vi "Move Motor.vi"(6 "Goal Speed (RPM)":dbl, 8 "error in (no error)":errorcluster, 9 "Goal Position (150 deg)":dbl=150.0 min=0.0 max=300.0, 10 "Motor ID (0)":u8, 11 "Dynamixel Motor Simulator in":refnum<class "Dynamixel Motor Simulator.lvclass">) -> (0 "error out":errorcluster, 3 "Dynamixel Motor Simulator out":refnum<class "Dynamixel Motor Simulator.lvclass">)   [LabVIEW 2016, in "Dynamixel Motor Simulator.lvclass"]
doc: "Sets the goal position for the motor."
uses:
  <instrlib>/Dynamixel Motor/HAIOL/Simulator/Dynamixel Motor Simulator.lvclass
  <instrlib>/Dynamixel Motor/HAIOL/Simulator/Dynamixel Motor Simulator.lvclass/Dynamixel Motor Simulator.ctl
  <vilib>/robotics/Simulator/Robot Factory/Motor/ODESimulator_Motor.lvclass
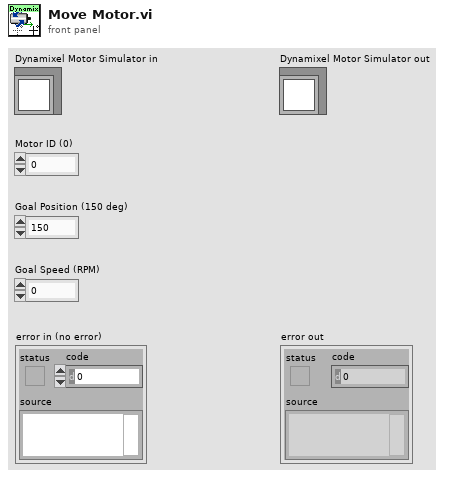
[diagram p1: front panel]
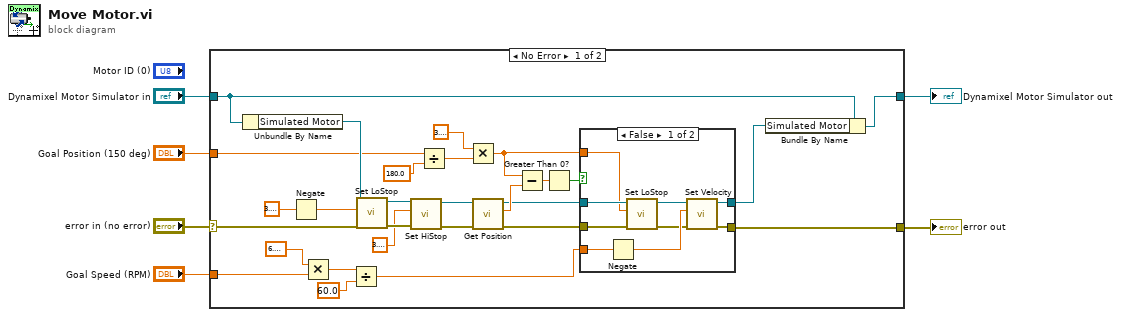
[diagram p0: block diagram]
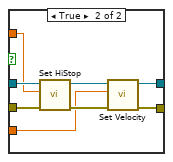
[diagram p2: hidden frame]
diagram:
  n1 = case shown="No Error" "error in (no error)" {
    selector: "error in (no error)" -> [w28 w52]
    tunnel: "Dynamixel Motor Simulator in" -> [w12 w53]
    tunnel: "Goal Speed (RPM)" -> [w33 _]
    tunnel: "Goal Position (150 deg)" -> [w18 _]
    tunnel: [w11 w53] -> w2
    tunnel: [w10 w52] -> w1
    frame No Error {
      n2 = Unbundle By Name(w12) -> ("Simulated Motor"=w25:refnum<class "ODESimulator_Motor.lvclass">)
      n3 = Negate(x=3.141592653589793) -> (-x=w7:dbl)
      n4 = Multiply(x=6.283185307179586, y=w33) -> (x*y=w32:dbl)
      n5 = Divide(x=w32, y=60.0) -> (x/y=w14:dbl)
      n6 = call-dynamic "Set LoStop.vi"("error in (no error)"=w28, "Lo Stop"=w7, "Motor in"=w25) -> ("error out"=w27:errorcluster, "Motor out"=w24:refnum<class "ODESimulator_Motor.lvclass">)  [unwired: 7 in]
      n7 = call-dynamic "Set HiStop.vi"("error in (no error)"=w27, "Hi Stop"=3.141592653589793, "Motor in"=w24) -> ("error out"=w26:errorcluster, "Motor out"=w23:refnum<class "ODESimulator_Motor.lvclass">)  [unwired: 7 in]
      n8 = Divide(x=w18, y=180.0) -> (x/y=w20:dbl)
      n9 = Multiply(x=3.141592653589793, y=w20) -> (x*y=w17:dbl)
      n10 = call-dynamic "Get Position.vi"("error in (no error)"=w26, "Motor in"=w23) -> ("error out"=w15:errorcluster, "CCW Position (rad)"=w30:dbl, "Motor out"=w16:refnum<class "ODESimulator_Motor.lvclass">)  [unwired: 7 in]
      n11 = Subtract(x=w17, y=w30) -> (x-y=w29:dbl)
      n12 = Greater Than 0?(x=w29) -> (x > 0?=w22:bool)
      n13 = case shown="False" w22 {
        tunnel: w17 -> [w37 w46]
        tunnel: w16 -> [w43 w51]
        tunnel: w15 -> [w42 w50]
        tunnel: w14 -> [w41 w47]
        tunnel: [w36 w45] -> w13
        tunnel: [w35 w44] -> w10
        frame False {
          n14 = Negate(x=w41) -> (-x=w40:dbl)
          n15 = call-dynamic "Set LoStop.vi"("error in (no error)"=w42, "Lo Stop"=w37, "Motor in"=w43) -> ("error out"=w38:errorcluster, "Motor out"=w39:refnum<class "ODESimulator_Motor.lvclass">)  [unwired: 7 in]
          n16 = call-dynamic "Set Velocity.vi"("error in (no error)"=w38, "CCW Velocity (0.0 rad/s)"=w40, "Motor in"=w39) -> ("error out"=w35:errorcluster, "Motor out"=w36:refnum<class "ODESimulator_Motor.lvclass">)  [unwired: 7 in]
        }
        frame True {
          n17 = call-dynamic "Set HiStop.vi"("error in (no error)"=w50, "Hi Stop"=w46, "Motor in"=w51) -> ("error out"=w48:errorcluster, "Motor out"=w49:refnum<class "ODESimulator_Motor.lvclass">)  [unwired: 7 in]
          n18 = call-dynamic "Set Velocity.vi"("error in (no error)"=w48, "CCW Velocity (0.0 rad/s)"=w47, "Motor in"=w49) -> ("error out"=w44:errorcluster, "Motor out"=w45:refnum<class "ODESimulator_Motor.lvclass">)  [unwired: 7 in]
        }
      }
      n19 = Bundle By Name(cluster=w12, "Simulated Motor"=w13) -> (w11:refnum<class "Dynamixel Motor Simulator.lvclass">)
    }
    frame Error {
    }
  }
  "error out" <- w1
  "Dynamixel Motor Simulator out" <- w2
